vi "rsscope_core_global.vi"() -> ()   [LabVIEW 2018] (continued)
"Help"="Returns the cell count.\n\nAvailable Repeated Capabilities:\nSerialBus: SB1, SB2, SB3, SB4\r\n\nRemote-control command(s):\nBUS<m>:CMSB:FRAMe<n>:CCOunt?"}, {"Level"=5, "Class Only"=FALSE, "Identifier"="RSSCOPE_ATTR_PROTOCOL_MANCHESTER_NRZ_ADD_CELL", "Descriptive Name"="Protocol Manchester NRZ Add Cell", "Data Type"=4, "Command"="BUS{SerialBus}:CMSB:FRAM<Frame>:APP", "Access"=1, "Range Table"="", "Read Callback"="", "Write Callback"="rsscope_FormatManchesterNRZFrameRepCapEvent_WriteCallback.vi", "Supported Models"="", "Instrument Options"="K50", "Flags"=0, "Help"="Creates an empty cell description and adds it to the end of the active frame description.\n\nAvailable Repeated Capabilities:\nSerialBus: SB1, SB2, SB3, SB4\r\n\nRemote-control command(s):\nBUS<m>:CMSB:FRAMe<n>:APPend"}, {"Level"=5, "Class Only"=FALSE, "Identifier"="RSSCOPE_ATTR_PROTOCOL_MANCHESTER_NRZ_CELL_NAME", "Descriptive Name"="Protocol Manchester NRZ Cell Name", "Data Type"=2, "Command"="BUS{SerialBus}:CMSB:FRAM<Frame>:CELL<Cell>:NAME", "Access"=2, "Range Table"="", "Read Callback"="rsscope_FormatManchesterNRZFrameRepCapString_ReadCallback.vi", "Write Callback"="rsscope_FormatManchesterNRZFrameRepCapString_WriteCallback.vi", "Supported Models"="", "Instrument Options"="K50", "Flags"=0, "Help"="Enables the user to set a cell name within a frame. Names do not have to be unique, they are just for user support.\n\nAvailable Repeated Capabilities:\nSerialBus: SB1, SB2, SB3, SB4\r\n\nRemote-control command(s):\nBUS<m>:CMSB:FRAMe<n>:CELL<o>:NAME"}, {"Level"=5, "Class Only"=FALSE, "Identifier"="RSSCOPE_ATTR_PROTOCOL_MANCHESTER_NRZ_CELL_BIT_COUNT", "Descriptive Name"="Protocol Manchester NRZ Cell Bit Count", "Data Type"=0, "Command"="BUS{SerialBus}:CMSB:FRAM<Frame>:CELL<Cell>:BITC", "Access"=2, "Range Table"="RsScope_rngManchesterNRZCellBitCount", "Read Callback"="rsscope_FormatManchesterNRZFrameRepCapInt32_ReadCallback.vi", "Write Callback"="rsscope_FormatManchesterNRZFrameRepCapInt32_WriteCallback.vi", "Supported Models"="", "Instrument Options"="K50", "Flags"=0, "Help"="Sets the bit count of a cell, hence its length. Based upon the lengths of the previous cells, this also defines the position of the cell start and end within a frame.\n\nAvailable Repeated Capabilities:\nSerialBus: SB1, SB2, SB3, SB4\r\n\nRemote-control command(s):\nBUS<m>:CMSB:FRAMe<n>:CELL<o>:BITCount"}, {"Level"=5, "Class Only"=FALSE, "Identifier"="RSSCOPE_ATTR_PROTOCOL_MANCHESTER_NRZ_CELL_CONDITION", "Descriptive Name"="Protocol Manchester NRZ Cell Condition", "Data Type"=2, "Command"="BUS{SerialBus}:CMSB:FRAM<Frame>:CELL<Cell>:COND", "Access"=2, "Range Table"="", "Read Callback"="rsscope_FormatManchesterNRZFrameRepCapString_ReadCallback.vi", "Write Callback"="rsscope_FormatManchesterNRZFrameRepCapString_WriteCallback.vi", "Supported Models"="", "Instrument Options"="K50", "Flags"=0, "Help"="Sets various operators for a cell, to identify, e.g., mandatory values such as a CRC checksum or an ID, that help to identify a frame. The implemented conditions and functionalities are the &apos;equal&apos; and &apos;array&apos; operators. The numeric format of the condition needs to be set according to RSSCOPE_ATTR_PROTOCOL_MANCHESTER_NRZ_CELL_FORMAT.\n\nAvailable Repeated Capabilities:\nSerialBus: SB1, SB2, SB3, SB4\r\n\nRemote-control command(s):\nBUS<m>:CMSB:FRAMe<n>:CELL<o>:CONDition"}, {"Level"=5, "Class Only"=FALSE, "Identifier"="RSSCOPE_ATTR_PROTOCOL_MANCHESTER_NRZ_CELL_FORMAT", "Descriptive Name"="Protocol Manchester NRZ Cell Format", "Data Type"=0, "Command"="BUS{SerialBus}:CMSB:FRAM<Frame>:CELL<Cell>:FORM", "Access"=2, "Range Table"="RsScope_rngNumericFormat", "Read Callback"="rsscope_FormatManchesterNRZFrameRepCapInt32_ReadCallback.vi", "Write Callback"="rsscope_FormatManchesterNRZFrameRepCapInt32_WriteCallback.vi", "Supported Models"="", "Instrument Options"="K50", "Flags"=0, "Help"="Selects the numeric data format for the RSSCOPE_ATTR_PROTOCOL_MANCHESTER_NRZ_CELL_CONDITION, as well as for the result and honeycomb display.\n\nAvailable Repeated Capabilities:\nSerialBus: SB1, SB2, SB3, SB4\r\n\nRemote-control command(s):\nBUS<m>:CMSB:FRAMe<n>:CELL<o>:FORMat"}, {"Level"=5, "Class Only"=FALSE, "Identifier"="RSSCOPE_ATTR_PROTOCOL_MANCHESTER_NRZ_CELL_BIT_ORDER", "Descriptive Name"="Protocol Manchester NRZ Cell Bit Order", "Data Type"=0, "Command"="BUS{SerialBus}:CMSB:FRAM<Frame>:CELL<Cell>:BIT", "Access"=2, "Range Table"="rsscope_rngBitOrder", "Read Callback"="rsscope_FormatManchesterNRZFrameRepCapInt32_ReadCallback.vi", "Write Callback"="rsscope_FormatManchesterNRZFrameRepCapInt32_WriteCallback.vi", "Supported Models"="", "Instrument Options"="K50", "Flags"=0, "Help"="Selects in which order the bits of a cell are evaluated, as well as presented in the results table and honeycomb display.\n\nAvailable Repeated Capabilities:\nSerialBus: SB1, SB2, SB3, SB4\r\n\nRemote-control command(s):\nBUS<m>:CMSB:FRAMe<n>:CELL<o>:BITorder"}, {"Level"=5, "Class Only"=FALSE, "Identifier"="RSSCOPE_ATTR_PROTOCOL_MANCHESTER_NRZ_CELL_COLOR", "Descriptive Name"="Protocol Manchester NRZ Cell Color", "Data Type"=0, "Command"="BUS{SerialBus}:CMSB:FRAM<Frame>:CELL<Cell>:COL", "Access"=2, "Range Table"="RsScope_rngCellColor", "Read Callback"="rsscope_FormatManchesterNRZFrameRepCapInt32_ReadCallback.vi", "Write Callback"="rsscope_FormatManchesterNRZFrameRepCapInt32_WriteCallback.vi", "Supported Models"="", "Instrument Options"="K50", "Flags"=0, "Help"="Selects a cell&apos;s color representation in the honeycomb display.\n\nAvailable Repeated Capabilities:\nSerialBus: SB1, SB2, SB3, SB4\r\n\nRemote-control command(s):\nBUS<m>:CMSB:FRAMe<n>:CELL<o>:COLor"}, {"Level"=5, "Class Only"=FALSE, "Identifier"="RSSCOPE_ATTR_PROTOCOL_MANCHESTER_NRZ_CELL_COLOR_CRGB", "Descriptive Name"="Protocol Manchester NRZ Cell Color CRGB", "Data Type"=5, "Command"="BUS{SerialBus}:CMSB:FRAM<Frame>:CELL<Cell>:CRGB", "Access"=2, "Range Table"="", "Read Callback"="rsscope_FormatManchesterNRZFrameRepCapInt64_ReadCallback.vi", "Write Callback"="rsscope_FormatManchesterNRZFrameRepCapInt64_WriteCallback.vi", "Supported Models"="", "Instrument Options"="K50", "Flags"=0, "Help"="Selects a cell&apos;s color representation in the honeycomb display. ARGB value of the color to be used for the table entry.\nARGB=<Opacity(alpha) value><red value><green value><blue value>, in decimal format.\n\nAvailable Repeated Capabilities:\nSerialBus: SB1, SB2, SB3, SB4\r\n\nRemote-control command(s):\nBUS<m>:CMSB:FRAMe<n>:CELL<o>:CRGB"}, {"Level"=5, "Class Only"=FALSE, "Identifier"="RSSCOPE_ATTR_PROTOCOL_MANCHESTER_NRZ_CELL_RESULT_COLUMN", "Descriptive Name"="Protocol Manchester NRZ Cell Result Column", "Data Type"=0, "Command"="BUS{SerialBus}:CMSB:FRAM<Frame>:CELL<Cell>:CLMN", "Access"=2, "Range Table"="RsScope_rngCellResultColumn", "Read Callback"="rsscope_FormatManchesterNRZFrameRepCapInt32_ReadCallback.vi", "Write Callback"="rsscope_FormatManchesterNRZFrameRepCapInt32_WriteCallback.vi", "Supported Models"="", "Instrument Options"="K50", "Flags"=0, "Help"="Selects which cell shall be displayed in which result column of the decode table. The decode table supports three result columns, which have to be unique for each frame type. For different frame types, though, different result columns can be defined to display unrelated information.\n\nAvailable Repeated Capabilities:\nSerialBus: SB1, SB2, SB3, SB4\r\n\nRemote-control command(s):\nBUS<m>:CMSB:FRAMe<n>:CELL<o>:CLMN"}, {"Level"=3, "Class Only"=TRUE, "Identifier"="", "Descriptive Name"="Filter", "Data Type"=0, "Command"="", "Access"=0, "Range Table"="", "Read Callback"="", "Write Callback"="", "Supported Models"="", "Instrument Options"="", "Flags"=0, "Help"="Configures filtering of custom serial bus."}, {"Level"=4, "Class Only"=FALSE, "Identifier"="RSSCOPE_ATTR_PROTOCOL_MANCHESTER_NRZ_SELECTED_FIELD", "Descriptive Name"="Protocol Manchester NRZ Selected Field", "Data Type"=0, "Command"="", "Access"=2, "Range Table"="", "Read Callback"="", "Write Callback"="", "Supported Models"="", "Instrument Options"="", "Flags"=0, "Help"="Sets the selector for the Field repeated capability.\n\nAvailable Repeated Capabilities:\nNone\n\nRemote-control command(s):\n"}, {"Level"=4, "Class Only"=FALSE, "Identifier"="RSSCOPE_ATTR_PROTOCOL_MANCHESTER_NRZ_FILTER_ENABLED", "Descriptive Name"="Protocol Manchester NRZ Filter Enabled", "Data Type"=3, "Command"="BUS{SerialBus}:CMSB:FILT:ENAB", "Access"=2, "Range Table"="", "Read Callback"="", "Write Callback"="", "Supported Models"="", "Instrument Options"="K50", "Flags"=0, "Help"="Enables filtering for the custom serial bus.\n\nAvailable Repeated Capabilities:\nSerialBus: SB1, SB2, SB3, SB4\r\n\nRemote-control command(s):\nBUS<m>:CMSB:FILTer:ENABle"}, {"Level"=4, "Class Only"=FALSE, "Identifier"="RSSCOPE_ATTR_PROTOCOL_MANCHESTER_NRZ_FILTER_FRAME_FIELD_NUMERIC_ENABLED", "Descriptive Name"="Protocol Manchester NRZ Filter Frame Field Numeric Enabled", "Data Type"=3, "Command"="BUS{SerialBus}:CMSB:FILT:FRAM<Frame>:FLD<Field>:ENAB", "Access"=2, "Range Table"="", "Read Callback"="rsscope_FormatManchesterNRZFrameFieldRepCapBoolean_ReadCallback.vi", "Write Callback"="rsscope_FormatManchesterNRZFrameFieldRepCapBoolean_WriteCallback.vi", "Supported Models"="", "Instrument Options"="", "Flags"=0, "Help"="Enables or disables the specific field within the defined frame to be filtered.\n\nAvailable Repeated Capabilities:\nSerialBus: SB1, SB2, SB3, SB4\r\n\nRemote-control command(s):\nBUS<m>:CMSB:FILTer:FRAMe<Frame>:FLD<Field>:ENABle"}, {"Level"=4, "Class Only"=FALSE, "Identifier"="RSSCOPE_ATTR_PROTOCOL_MANCHESTER_NRZ_FILTER_FRAME_FIELD_BIT_STATE", "Descriptive Name"="Protocol Manchester NRZ Filter Frame Field Bit State", "Data Type"=0, "Command"="BUS{SerialBus}:CMSB:FILT:FRAM<Frame>:FLD<Field>:BIT", "Access"=2, "Range Table"="RsScope_rngBitState", "Read Callback"="rsscope_FormatManchesterNRZFrameFieldRepCapInt32_ReadCallback.vi", "Write Callback"="rsscope_FormatManchesterNRZFrameFieldRepCapInt32_WriteCallback.vi", "Supported Models"="", "Instrument Options"="", "Flags"=0, "Help"="Sets the bit state of a field to be filtered on that only consists of one bit.\n\nAvailable Repeated Capabilities:\nSerialBus: SB1, SB2, SB3, SB4\r\n\nRemote-control command(s):\nBUS<m>:CMSB:FILTer:FRAMe<n>:FLD<o>:BIT"}, {"Level"=4, "Class Only"=FALSE, "Identifier"="RSSCOPE_ATTR_PROTOCOL_MANCHESTER_NRZ_FILTER_FRAME_FIELD_DATA_PATTERN_CONDITION", "Descriptive Name"="Protocol Manchester NRZ Filter Frame Field Data Pattern Condition", "Data Type"=0, "Command"="BUS{SerialBus}:CMSB:FILT:FRAM<Frame>:FLD<Field>:DOP", "Access"=2, "Range Table"="rsscope_rngCustomSBCondition", "Read Callback"="rsscope_FormatManchesterNRZFrameFieldRepCapInt32_ReadCallback.vi", "Write Callback"="rsscope_FormatManchesterNRZFrameFieldRepCapInt32_WriteCallback.vi", "Supported Models"="", "Instrument Options"="", "Flags"=0, "Help"="Sets the operator for the data pattern.\n\nAvailable Repeated Capabilities:\nSerialBus: SB1, SB2, SB3, SB4\r\n\nRemote-control command(s):\nBUS<m>:CMSB:FILTer:FRAMe<n>:FLD<o>:DOPerator"}, {"Level"=4, "Class Only"=FALSE, "Identifier"="RSSCOPE_ATTR_PROTOCOL_MANCHESTER_NRZ_FILTER_FRAME_FIELD_DATA_PATTERN_MIN", "Descriptive Name"="Protocol Manchester NRZ Filter Frame Field Data Pattern Min", "Data Type"=6, "Command"="BUS{SerialBus}:CMSB:FILT:FRAM<Frame>:FLD<Field>:DMIN", "Access"=2, "Range Table"="", "Read Callback"="rsscope_FormatManchesterNRZFrameFieldRepCapRawString_ReadCallback.vi", "Write Callback"="rsscope_FormatManchesterNRZFrameFieldRepCapRawString_WriteCallback.vi", "Supported Models"="", "Instrument Options"="", "Flags"=0, "Help"="Specifies the data pattern, or sets the start value of a data pattern range.\n\nAvailable Repeated Capabilities:\nSerialBus: SB1, SB2, SB3, SB4\r\n\nRemote-control command(s):\nBUS<m>:CMSB:FILTer:FRAMe<n>:FLD<o>:DMIN"}, {"Level"=4, "Class Only"=FALSE, "Identifier"="RSSCOPE_ATTR_PROTOCOL_MANCHESTER_NRZ_FILTER_FRAME_FIELD_DATA_PATTERN_MAX", "Descriptive Name"="Protocol Manchester NRZ Filter Frame Field Data Pattern Max", "Data Type"=6, "Command"="BUS{SerialBus}:CMSB:FILT:FRAM<Frame>:FLD<Field>:DMAX", "Access"=2, "Range Table"="", "Read Callback"="rsscope_FormatManchesterNRZFrameFieldRepCapRawString_ReadCallback.vi", "Write Callback"="rsscope_FormatManchesterNRZFrameFieldRepCapRawString_WriteCallback.vi", "Supported Models"="", "Instrument Options"="", "Flags"=0, "Help"="Sets the end value of a data pattern range if RSSCOPE_ATTR_PROTOCOL_MANCHESTER_NRZ_FILTER_FRAME_FIELD_DATA_PATTERN_CONDITION is set to In Range or Out Of Range.\n\nAvailable Repeated Capabilities:\nSerialBus: SB1, SB2, SB3, SB4\r\n\nRemote-control command(s):\nBUS<m>:CMSB:FILTer:FRAMe<n>:FLD<o>:DMAX"}, {"Level"=4, "Class Only"=FALSE, "Identifier"="RSSCOPE_ATTR_PROTOCOL_MANCHESTER_NRZ_FILTER_FRAME_FIELD_INDEX_PATTERN_CONDITION", "Descriptive Name"="Protocol Manchester NRZ Filter Frame Field Index Pattern Condition", "Data Type"=0, "Command"="BUS{SerialBus}:CMSB:FILT:FRAM<Frame>:FLD<Field>:IOP", "Access"=2, "Range Table"="rsscope_rngCustomSBCondition", "Read Callback"="rsscope_FormatManchesterNRZFrameFieldRepCapInt32_ReadCallback.vi", "Write Callback"="rsscope_FormatManchesterNRZFrameFieldRepCapInt32_WriteCallback.vi", "Supported Models"="", "Instrument Options"="", "Flags"=0, "Help"="Sets the operator for the index in the selected field of the selected frame.\n\nAvailable Repeated Capabilities:\nSerialBus: SB1, SB2, SB3, SB4\r\n\nRemote-control command(s):\nBUS<m>:CMSB:FILTer:FRAMe<n>:FLD<o>:IOPerator"}, {"Level"=4, "Class Only"=FALSE, "Identifier"="RSSCOPE_ATTR_PROTOCOL_MANCHESTER_NRZ_FILTER_FRAME_FIELD_INDEX_PATTERN_MIN", "Descriptive Name"="Protocol Manchester NRZ Filter Frame Field Index Pattern Min", "Data Type"=6, "Command"="BUS{SerialBus}:CMSB:FILT:FRAM<Frame>:FLD<Field>:IMIN", "Access"=2, "Range Table"="", "Read Callback"="rsscope_FormatManchesterNRZFrameFieldRepCapRawString_ReadCallback.vi", "Write Callback"="rsscope_FormatManchesterNRZFrameFieldRepCapRawString_WriteCallback.vi", "Supported Models"="", "Instrument Options"="", "Flags"=0, "Help"="Specifies the index, or sets the start value of an index range.\n\nAvailable Repeated Capabilities:\nSerialBus: SB1, SB2, SB3, SB4\r\n\nRemote-control command(s):\nBUS<m>:CMSB:FILTer:FRAMe<n>:FLD<o>:IMIN"}, {"Level"=4, "Class Only"=FALSE, "Identifier"="RSSCOPE_ATTR_PROTOCOL_MANCHESTER_NRZ_FILTER_FRAME_FIELD_INDEX_PATTERN_MAX", "Descriptive Name"="Protocol Manchester NRZ Filter Frame Field Index Pattern Max", "Data Type"=6, "Command"="BUS{SerialBus}:CMSB:FILT:FRAM<Frame>:FLD<Field>:IMAX", "Access"=2, "Range Table"="", "Read Callback"="rsscope_FormatManchesterNRZFrameFieldRepCapRawString_ReadCallback.vi", "Write Callback"="rsscope_FormatManchesterNRZFrameFieldRepCapRawString_WriteCallback.vi", "Supported Models"="", "Instrument Options"="", "Flags"=0, "Help"="Sets the end value of a index pattern range if RSSCOPE_ATTR_PROTOCOL_MANCHESTER_NRZ_FILTER_FRAME_FIELD_INDEX_PATTERN_CONDITION is set to In Range or Out Of Range.\n\nAvailable Repeated Capabilities:\nSerialBus: SB1, SB2, SB3, SB4\r\n\nRemote-control command(s):\nBUS<m>:CMSB:FILTer:FRAMe<n>:FLD<o>:IMAX"}, {"Level"=3, "Class Only"=TRUE, "Identifier"="", "Descriptive Name"="Decoding Results", "Data Type"=0, "Command"="", "Access"=0, "Range Table"="", "Read Callback"="", "Write Callback"="", "Supported Models"="", "Instrument Options"="", "Flags"=0, "Help"="Returns the decoding results."}, {"Level"=4, "Class Only"=FALSE, "Identifier"="RSSCOPE_ATTR_PROTOCOL_MANCHESTER_NRZ_RESULT_COUNT", "Descriptive Name"="Protocol Manchester NRZ Result Count", "Data Type"=0, "Command"="BUS{SerialBus}:CMSB:RCO?", "Access"=0, "Range Table"="", "Read Callback"="", "Write Callback"="", "Supported Models"="", "Instrument Options"="K50", "Flags"=0, "Help"="Returns the count number of decoded result frames in a custom serial bus waveform.\n\nAvailable Repeated Capabilities:\nSerialBus: SB1, SB2, SB3, SB4\r\n\nRemote-control command(s):\nBUS<m>:CMSB:RCOunt?"}, {"Level"=2, "Class Only"=TRUE, "Identifier"="", "Descriptive Name"="EbTb", "Data Type"=0, "Command"="", "Access"=0, "Range Table"="", "Read Callback"="", "Write Callback"="", "Supported Models"="", "Instrument Options"="", "Flags"=0, "Help"="The 8b/10b (Option R&S RTO-K52) coding scheme is used for high-speed serial data transmission, used by different standards, like fibre channel, PCIe, DVI and USB 3.0. Also the MIPI UniPro M-PHY interface in smartphones as well as display interfaces such as HDMI use 8b/10b encoding, as do base stations based on the Common Public Radio Interface (CPRI)."}, {"Level"=3, "Class Only"=FALSE, "Identifier"="RSSCOPE_ATTR_PROTOCOLS_EBTB_SIGNAL_TYPE", "Descriptive Name"="Protocols EbTb Signal Type", "Data Type"=0, "Command"="BUS{SerialBus}:EBTB:TYPE", "Access"=2, "Range Table"="RsScope_rngSignalType", "Read Callback"="", "Write Callback"="", "Supported Models"="", "Instrument Options"="K52", "Flags"=0, "Help"="Selects the signal type that is used for the decoding. You can choose between a differential and single-ended signal.\n\nAvailable Repeated Capabilities:\nSerialBus: SB1, SB2, SB3, SB4\r\n\nRemote-control command(s):\nBUS<m>:EBTB:TYPE"}, {"Level"=3, "Class Only"=FALSE, "Identifier"="RSSCOPE_ATTR_PROTOCOLS_EBTB_DIFFERENTIAL_SOURCE", "Descriptive Name"="Protocols EbTb Differential Source", "Data Type"=0, "Command"="BUS{SerialBus}:EBTB:DIFF:SOUR", "Access"=2, "Range Table"="rsscope_rngWaveformParameter", "Read Callback"="", "Write Callback"="", "Supported Models"="", "Instrument Options"="K52", "Flags"=0, "Help"="Selects the source of the provided differential signal, if 'Signal type' > 'Differential'.\n\nAvailable Repeated Capabilities:\nSerialBus: SB1, SB2, SB3, SB4\r\n\nRemote-control command(s):\nBUS<m>:EBTB:DIFFerential:SOURce"}, {"Level"=3, "Class Only"=FALSE, "Identifier"="RSSCOPE_ATTR_PROTOCOLS_EBTB_D_PLUS_SOURCE", "Descriptive Name"="Protocols EbTb D Plus Source", "Data Type"=0, "Command"="BUS{SerialBus}:EBTB:DPL:SOUR", "Access"=2, "Range Table"="rsscope_rngWaveformParameter", "Read Callback"="", "Write Callback"="", "Supported Models"="", "Instrument Options"="K52", "Flags"=0, "Help"="Selects the D+ source of the provided single-ended signal, if 'Signal type' > 'Single.\n\nAvailable Repeated Capabilities:\nSerialBus: SB1, SB2, SB3, SB4\r\n\nRemote-control command(s):\nBUS<m>:EBTB:DPLus:SOURce"}, {"Level"=3, "Class Only"=FALSE, "Identifier"="RSSCOPE_ATTR_PROTOCOLS_EBTB_D_MINUS_SOURCE", "Descriptive Name"="Protocols EbTb D Minus Source", "Data Type"=0, "Command"="BUS{SerialBus}:EBTB:DMIN:SOUR", "Access"=2, "Range Table"="rsscope_rngWaveformParameter", "Read Callback"="", "Write Callback"="", "Supported Models"="", "Instrument Options"="K52", "Flags"=0, "Help"="Selects the D- source of the provided single ended signal, if 'Signal type' > 'Single\n\nAvailable Repeated Capabilities:\nSerialBus: SB1, SB2, SB3, SB4\r\n\nRemote-control command(s):\nBUS<m>:EBTB:DMINus:SOURce"}, {"Level"=3, "Class Only"=FALSE, "Identifier"="RSSCOPE_ATTR_PROTOCOLS_EBTB_FULL_AUTOSET", "Descriptive Name"="Protocols EbTb Full Autoset", "Data Type"=4, "Command"="BUS{SerialBus}:EBTB:FAUT", "Access"=1, "Range Table"="", "Read Callback"="", "Write Callback"="", "Supported Models"="", "Instrument Options"="K52", "Flags"=0, "Help"="Starts software algorithms for determining the signal threshold levels and bitrate.\n\nAvailable Repeated Capabilities:\nSerialBus: SB1, SB2, SB3, SB4\r\n\nRemote-control command(s):\nBUS<m>:EBTB:FAUToscale"}, {"Level"=3, "Class Only"=FALSE, "Identifier"="RSSCOPE_ATTR_PROTOCOLS_EBTB_DIFFERENTIAL_THRESHOLD_HIGH", "Descriptive Name"="Protocols EbTb Differential Threshold High", "Data Type"=1, "Command"="BUS{SerialBus}:EBTB:DIFF:THRH", "Access"=2, "Range Table"="RsScope_rngEbTbThreshold", "Read Callback"="", "Write Callback"="", "Supported Models"="", "Instrument Options"="K52", "Flags"=0, "Help"="Sets the threshold high of the signal, if &apos;Signal type&apos; > &apos;Differential&apos;.\n\nAvailable Repeated Capabilities:\nSerialBus: SB1, SB2, SB3, SB4\r\n\nRemote-control command(s):\nBUS<m>:EBTB:DIFFerential:THRHigh"}, {"Level"=3, "Class Only"=FALSE, "Identifier"="RSSCOPE_ATTR_PROTOCOLS_EBTB_DIFFERENTIAL_THRESHOLD_LOW", "Descriptive Name"="Protocols EbTb Differential Threshold Low", "Data Type"=1, "Command"="BUS{SerialBus}:EBTB:DIFF:THRL", "Access"=2, "Range Table"="RsScope_rngEbTbThreshold", "Read Callback"="", "Write Callback"="", "Supported Models"="", "Instrument Options"="K52", "Flags"=0, "Help"="Sets the threshold low of the signal, if &apos;Signal type&apos; > &apos;Differential&apos;.\n\nAvailable Repeated Capabilities:\nSerialBus: SB1, SB2, SB3, SB4\r\n\nRemote-control command(s):\nBUS<m>:EBTB:DIFFerential:THRLow"}, {"Level"=3, "Class Only"=FALSE, "Identifier"="RSSCOPE_ATTR_PROTOCOLS_EBTB_THRESHOLD_D_PLUS", "Descriptive Name"="Protocols EbTb Threshold D Plus", "Data Type"=1, "Command"="BUS{SerialBus}:EBTB:DPL:THR", "Access"=2, "Range Table"="RsScope_rngEbTbThreshold", "Read Callback"="", "Write Callback"="", "Supported Models"="", "Instrument Options"="K52", "Flags"=0, "Help"="Sets the high threshold (D+) of the signal, if &apos;Signal type&apos; > &apos;Single&apos;.\n\nAvailable Repeated Capabilities:\nSerialBus: SB1, SB2, SB3, SB4\r\n\nRemote-control command(s):\nBUS<m>:EBTB:DPLus:THReshold"}, {"Level"=3, "Class Only"=FALSE, "Identifier"="RSSCOPE_ATTR_PROTOCOLS_EBTB_THRESHOLD_D_MINUS", "Descriptive Name"="Protocols EbTb Threshold D Minus", "Data Type"=1, "Command"="BUS{SerialBus}:EBTB:DMIN:THR", "Access"=2, "Range Table"="RsScope_rngEbTbThreshold", "Read Callback"="", "Write Callback"="", "Supported Models"="", "Instrument Options"="K52", "Flags"=0, "Help"="Sets the low threshold (D-) of the signal, if &apos;Signal type&apos; > &apos;Single&apos;.\n\nAvailable Repeated Capabilities:\nSerialBus: SB1, SB2, SB3, SB4\r\n\nRemote-control command(s):\nBUS<m>:EBTB:DMINus:THReshold"}, {"Level"=3, "Class Only"=FALSE, "Identifier"="RSSCOPE_ATTR_PROTOCOLS_EBTB_BITRATE", "Descriptive Name"="Protocols EbTb Bitrate", "Data Type"=1, "Command"="BUS{SerialBus}:EBTB:BITR", "Access"=2, "Range Table"="RsScope_rngEbTbBitrate", "Read Callback"="", "Write Callback"="", "Supported Models"="", "Instrument Options"="K52", "Flags"=0, "Help"="Sets the number of transmitted bits per second.\n\nAvailable Repeated Capabilities:\nSerialBus: SB1, SB2, SB3, SB4\r\n\nRemote-control command(s):\nBUS<m>:EBTB:BITRate"}, {"Level"=3, "Class Only"=FALSE, "Identifier"="RSSCOPE_ATTR_PROTOCOLS_EBTB_BITRATE_DETERMINATION", "Descriptive Name"="Protocols EbTb Bitrate Determination", "Data Type"=4, "Command"="BUS{SerialBus}:EBTB:BITD", "Access"=1, "Range Table"="", "Read Callback"="", "Write Callback"="", "Supported Models"="", "Instrument Options"="K52", "Flags"=0, "Help"="Starts a software algorithm for the automatic determination of the bitrate.\n\nAvailable Repeated Capabilities:\nSerialBus: SB1, SB2, SB3, SB4\r\n\nRemote-control command(s):\nBUS<m>:EBTB:BITDetermi"}, {"Level"=3, "Class Only"=FALSE, "Identifier"="RSSCOPE_ATTR_PROTOCOLS_EBTB_ESTIMATED_BITRATE", "Descriptive Name"="Protocols EbTb Estimated Bitrate", "Data Type"=1, "Command"="BUS{SerialBus}:EBTB:EBTR?", "Access"=0, "Range Table"="", "Read Callback"="", "Write Callback"="", "Supported Models"="", "Instrument Options"="K52", "Flags"=0, "Help"="Queries the estimated bitrate value.\n\nAvailable Repeated Capabilities:\nSerialBus: SB1, SB2, SB3, SB4\r\n\nRemote-control command(s):\nBUS<m>:EBTB:EBTRate?"}, {"Level"=3, "Class Only"=FALSE, "Identifier"="RSSCOPE_ATTR_PROTOCOLS_EBTB_SW_CDR_BITRATE", "Descriptive Name"="Protocols EbTb SW CDR Bitrate", "Data Type"=3, "Command"="BUS{SerialBus}:EBTB:ACT", "Access"=2, "Range Table"="", "Read Callback"="", "Write Callback"="", "Supported Models"="", "Instrument Options"="K52", "Flags"=0, "Help"="Disables the automatic software birtate determination.\n\nAvailable Repeated Capabilities:\nSerialBus: SB1, SB2, SB3, SB4\r\n\nRemote-control command(s):\nBUS<m>:EBTB:ACTestimate"}, {"Level"=3, "Class Only"=FALSE, "Identifier"="RSSCOPE_ATTR_PROTOCOLS_EBTB_SYNC_SYMBOL", "Descriptive Name"="Protocols EbTb Sync Symbol", "Data Type"=0, "Command"="BUS{SerialBus}:EBTB:SYNC", "Access"=2, "Range Table"="RsScope_rngEbTbSyncSymbol", "Read Callback"="", "Write Callback"="", "Supported Models"="", "Instrument Options"="K52", "Flags"=0, "Help"="Selects the sync symbol, a control symbol used for low level control functions. You can select one of the comma control symbols (K28.1, K28.5, K28.7) used for synchronisation or you can enter a pattern.\n\nAvailable Repeated Capabilities:\nSerialBus: SB1, SB2, SB3, SB4\r\n\nRemote-control command(s):\nBUS<m>:EBTB:SYNC"}, {"Level"=3, "Class Only"=FALSE, "Identifier"="RSSCOPE_ATTR_PROTOCOLS_EBTB_PATTERN", "Descriptive Name"="Protocols EbTb Pattern", "Data Type"=0, "Command"="BUS{SerialBus}:EBTB:FCSY", "Access"=2, "Range Table"="", "Read Callback"="", "Write Callback"="", "Supported Models"="", "Instrument Options"="K52", "Flags"=0, "Help"="Selects a pattern that serves as a sync symbol.\n\nAvailable Repeated Capabilities:\nSerialBus: SB1, SB2, SB3, SB4\r\n\nRemote-control command(s):\nBUS<m>:EBTB:FCSY"}, {"Level"=3, "Class Only"=FALSE, "Identifier"="RSSCOPE_ATTR_PROTOCOLS_EBTB_SECOND_PATTERN_ENABLED", "Descriptive Name"="Protocols EbTb Second Pattern Enabled", "Data Type"=3, "Command"="BUS{SerialBus}:EBTB:USCS", "Access"=2, "Range Table"="", "Read Callback"="", "Write Callback"="", "Supported Models"="", "Instrument Options"="K52", "Flags"=0, "Help"="Selects whether the second pattern is enabled.\n\nAvailable Repeated Capabilities:\nSerialBus: SB1, SB2, SB3, SB4\r\n\nRemote-control command(s):\nBUS<m>:EBTB:USCS"}, {"Level"=3, "Class Only"=FALSE, "Identifier"="RSSCOPE_ATTR_PROTOCOLS_EBTB_SECOND_PATTERN", "Descriptive Name"="Protocols EbTb Second Pattern", "Data Type"=0, "Command"="BUS{SerialBus}:EBTB:SCSY", "Access"=2, "Range Table"="", "Read Callback"="", "Write Callback"="", "Supported Models"="", "Instrument Options"="K52", "Flags"=0, "Help"="Sets the value for the second pattern.\n\nAvailable Repeated Capabilities:\nSerialBus: SB1, SB2, SB3, SB4\r\n\nRemote-control command(s):\nBUS<m>:EBTB:SCSY"}, {"Level"=3, "Class Only"=FALSE, "Identifier"="RSSCOPE_ATTR_PROTOCOLS_EBTB_DISPLAY_FORMAT", "Descriptive Name"="Protocols EbTb Display Format", "Data Type"=0, "Command"="BUS{SerialBus}:EBTB:DISF", "Access"=2, "Range Table"="RsScope_rngEbTbDisplayFormat", "Read Callback"="", "Write Callback"="", "Supported Models"="", "Instrument Options"="K52", "Flags"=0, "Help"="Selects the display format for the results in the decode table.\n\nAvailable Repeated Capabilities:\nSerialBus: SB1, SB2, SB3, SB4\r\n\nRemote-control command(s):\nBUS<m>:EBTB:DISF"}, {"Level"=3, "Class Only"=TRUE, "Identifier"="", "Descriptive Name"="Decoding Results", "Data Type"=0, "Command"="", "Access"=0, "Range Table"="", "Read Callback"="", "Write Callback"="", "Supported Models"="", "Instrument Options"="", "Flags"=0, "Help"="Returns the decoding results."}, {"Level"=4, "Class Only"=FALSE, "Identifier"="RSSCOPE_ATTR_PROTOCOL_EBTB_SYMBOL_COUNT", "Descriptive Name"="Protocol EbTb Symbol Count", "Data Type"=0, "Command"="BUS{SerialBus}:EBTB:SCO?", "Access"=0, "Range Table"="", "Read Callback"="", "Write Callback"="", "Supported Models"="", "Instrument Options"="K52", "Flags"=0, "Help"="Returns the symbol count for the selected serial bus, i.e. the number of symbols in the present acquisition.\n\nAvailable Repeated Capabilities:\nSerialBus: SB1, SB2, SB3, SB4\r\n\nRemote-control command(s):\nBUS<m>:EBTB:SCOunt?"}, {"Level"=2, "Class Only"=TRUE, "Identifier"="", "Descriptive Name"="SENT", "Data Type"=0, "Command"="", "Access"=0, "Range Table"="", "Read Callback"="", "Write Callback"="", "Supported Models"="", "Instrument Options"="", "Flags"=0, "Help"="SENT (Single Ended Nibble Transmission, R&S RTO-K10 option) is a serial transmission interface protocol originally specified for the communication of sensors and control units in automotive electronics."}, {"Level"=3, "Class Only"=FALSE, "Identifier"="RSSCOPE_ATTR_PROTOCOL_SENT_DATA_SOURCE", "Descriptive Name"="Protocol SENT Data Source", "Data Type"=0, "Command"="BUS{SerialBus}:SENT:DATA:SOUR", "Access"=2, "Range Table"="rsscope_rngProtocolWaveformSource", "Read Callback"="", "Write Callback"="", "Supported Models"="", "Instrument Options"="K10", "Flags"=0, "Help"="Selects the source of the data line.\n\nAvailable Repeated Capabilities:\nSerialBus: SB1, SB2, SB3, SB4\r\n\nRemote-control command(s):\nBUS<m>:SENT:DATA:SOURce"}, {"Level"=3, "Class Only"=FALSE, "Identifier"="RSSCOPE_ATTR_PROTOCOL_SENT_THRESHOLD", "Descriptive Name"="Protocol SENT Threshold", "Data Type"=1, "Command"="BUS{SerialBus}:SENT:DATA:THR", "Access"=2, "Range Table"="RsScope_rngSENTThreshold", "Read Callback"="", "Write Callback"="", "Supported Models"="", "Instrument Options"="K10", "Flags"=0, "Help"="Sets a user-defined threshold value.\n\nAvailable Repeated Capabilities:\nSerialBus: SB1, SB2, SB3, SB4\r\n\nRemote-control command(s):\nBUS<m>:SENT:DATA:THReshold"}, {"Level"=3, "Class Only"=FALSE, "Identifier"="RSSCOPE_ATTR_PROTOCOL_SENT_TECHNOLOGY", "Descriptive Name"="Protocol SENT Technology", "Data Type"=0, "Command"="BUS{SerialBus}:SENT:TECH", "Access"=2, "Range Table"="RsScope_rngSENTTechnology", "Read Callback"="", "Write Callback"="", "Supported Models"="", "Instrument Options"="K10", "Flags"=0, "Help"="Selects the threshold voltage.\n\nAvailable Repeated Capabilities:\nSerialBus: SB1, SB2, SB3, SB4\r\n\nRemote-control command(s):\nBUS<m>:SENT:TECHnology"}, {"Level"=3, "Class Only"=FALSE, "Identifier"="RSSCOPE_ATTR_PROTOCOL_SENT_CLOCK_PERIOD", "Descriptive Name"="Protocol SENT Clock Period", "Data Type"=1, "Command"="BUS{SerialBus}:SENT:CLKP", "Access"=2, "Range Table"="RsScope_rngSENTClockPeriod", "Read Callback"="", "Write Callback"="", "Supported Models"="", "Instrument Options"="K10", "Flags"=0, "Help"="Sets the nominal clock period (clock tick).\n\nAvailable Repeated Capabilities:\nSerialBus: SB1, SB2, SB3, SB4\r\n\nRemote-control command(s):\nBUS<m>:SENT:CLKPeriod"}, {"Level"=3, "Class Only"=FALSE, "Identifier"="RSSCOPE_ATTR_PROTOCOL_SENT_CLOCK_TOLERANCE", "Descriptive Name"="Protocol SENT Clock Tolerance", "Data Type"=1, "Command"="BUS{SerialBus}:SENT:CLKT", "Access"=2, "Range Table"="RsScope_rngSENTClockTolerance", "Read Callback"="", "Write Callback"="", "Supported Models"="", "Instrument Options"="K10", "Flags"=0, "Help"="Specifies a tolerated deviation of the clock.\n\nAvailable Repeated Capabilities:\nSerialBus: SB1, SB2, SB3, SB4\r\n\nRemote-control command(s):\nBUS<m>:SENT:CLKTolerance"}, {"Level"=3, "Class Only"=FALSE, "Identifier"="RSSCOPE_ATTR_PROTOCOL_SENT_DATA_NIBBLES", "Descriptive Name"="Protocol SENT Data Nibbles", "Data Type"=0, "Command"="BUS{SerialBus}:SENT:DNIB", "Access"=2, "Range Table"="RsScope_rngSENTDataNibbles", "Read Callback"="", "Write Callback"="", "Supported Models"="", "Instrument Options"="K10", "Flags"=0, "Help"="Sets the number of data nibbles for a transmission sequence.\n\nAvailable Repeated Capabilities:\nSerialBus: SB1, SB2, SB3, SB4\r\n\nRemote-control command(s):\nBUS<m>:SENT:DNIBbles"}, {"Level"=3, "Class Only"=FALSE, "Identifier"="RSSCOPE_ATTR_PROTOCOL_SENT_SERIAL_FORMAT", "Descriptive Name"="Protocol SENT Serial Format", "Data Type"=0, "Command"="BUS{SerialBus}:SENT:SFOR", "Access"=2, "Range Table"="RsScope_rngSENTSerialFormat", "Read Callback"="", "Write Callback"="", "Supported Models"="", "Instrument Options"="K10", "Flags"=0, "Help"="Selects the serial message format.\n\nAvailable Repeated Capabilities:\nSerialBus: SB1, SB2, SB3, SB4\r\n\nRemote-control command(s):\nBUS<m>:SENT:SFORmat"}, {"Level"=3, "Class Only"=FALSE, "Identifier"="RSSCOPE_ATTR_PROTOCOL_SENT_CRC_VERSION", "Descriptive Name"="Protocol SENT CRC Version", "Data Type"=0, "Command"="BUS{SerialBus}:SENT:CRCV", "Access"=2, "Range Table"="RsScope_rngSENTCRCVersion", "Read Callback"="", "Write Callback"="", "Supported Models"="", "Instrument Options"="K10", "Flags"=0, "Help"="Selects the calculaction method for the cyclic redundancy check (CRC).\n\nAvailable Repeated Capabilities:\nSerialBus: SB1, SB2, SB3, SB4\r\n\nRemote-control command(s):\nBUS<m>:SENT:CRCVersion"}, {"Level"=3, "Class Only"=FALSE, "Identifier"="RSSCOPE_ATTR_PROTOCOL_SENT_CRC_CALCULATION", "Descriptive Name"="Protocol SENT CRC Calculation", "Data Type"=0, "Command"="BUS{SerialBus}:SENT:CRCM", "Access"=2, "Range Table"="RsScope_rngSENTCRCMethod", "Read Callback"="", "Write Callback"="", "Supported Models"="", "Instrument Options"="K10", "Flags"=0, "Help"="Selects the method for CRC calculation. SENT CRC calculates the checksum over all nibbles except the communication and\nstatus nibble.\n\nAvailable Repeated Capabilities:\nSerialBus: SB1, SB2, SB3, SB4\r\n\nRemote-control command(s):\nBUS<m>:SENT:CRCMethod"}, {"Level"=3, "Class Only"=FALSE, "Identifier"="RSSCOPE_ATTR_PROTOCOL_SENT_PAUSE_PULSE", "Descriptive Name"="Protocol SENT Pause Pulse", "Data Type"=0, "Command"="BUS{SerialBus}:SENT:PPUL", "Access"=2, "Range Table"="RsScope_rngSENTPausePulse", "Read Callback"="", "Write Callback"="", "Supported Models"="", "Instrument Options"="K10", "Flags"=0, "Help"="Determines wether a pause pulse is part of the SENT transmission sequence.\n\nAvailable Repeated Capabilities:\nSerialBus: SB1, SB2, SB3, SB4\r\n\nRemote-control command(s):\nBUS<m>:SENT:PPULse"}, {"Level"=3, "Class Only"=FALSE, "Identifier"="RSSCOPE_ATTR_PROTOCOL_SENT_FRAME_LENGTH", "Descriptive Name"="Protocol SENT Frame Length", "Data Type"=0, "Command"="BUS{SerialBus}:SENT:PPFL", "Access"=2, "Range Table"="RsScope_rngSENTFrameLength", "Read Callback"="", "Write Callback"="", "Supported Models"="", "Instrument Options"="K10", "Flags"=0, "Help"="Determines the frame length in terms of ticks. The dialog displays this settings parameter, if the signal has a constant frame length.\n\nAvailable Repeated Capabilities:\nSerialBus: SB1, SB2, SB3, SB4\r\n\nRemote-control command(s):\nBUS<m>:SENT:PPFLength"}, {"Level"=3, "Class Only"=FALSE, "Identifier"="RSSCOPE_ATTR_PROTOCOL_SENT_RESULT_DISPLAY", "Descriptive Name"="Protocol SENT Result Display", "Data Type"=0, "Command"="BUS{SerialBus}:SENT:RDSL", "Access"=2, "Range Table"="RsScope_rngSENTResultDisplay", "Read Callback"="", "Write Callback"="", "Supported Models"="", "Instrument Options"="K10", "Flags"=0, "Help"="Selects the results to be displayed.\n\nAvailable Repeated Capabilities:\nSerialBus: SB1, SB2, SB3, SB4\r\n\nRemote-control command(s):\nBUS<m>:SENT:RDSL"}, {"Level"=3, "Class Only"=TRUE, "Identifier"="", "Descriptive Name"="Decoding Results", "Data Type"=0, "Command"="", "Access"=0, "Range Table"="", "Read Callback"="", "Write Callback"="", "Supported Models"="", "Instrument Options"="", "Flags"=0, "Help"="Returns the decoding results."}, {"Level"=4, "Class Only"=FALSE, "Identifier"="RSSCOPE_ATTR_PROTOCOL_SENT_FRAME_COUNT", "Descriptive Name"="Protocol SENT Frame Count", "Data Type"=0, "Command"="BUS{SerialBus}:SENT:FCO?", "Access"=0, "Range Table"="", "Read Callback"="", "Write Callback"="", "Supported Models"="", "Instrument Options"="K10", "Flags"=0, "Help"="Returns the number of decoded frames of the acquisition.\n\nAvailable Repeated Capabilities:\nSerialBus: SB1, SB2, SB3, SB4\r\n\nRemote-control command(s):\nBUS<m>:SENT:FCOunt?"}, {"Level"=2, "Class Only"=TRUE, "Identifier"="", "Descriptive Name"="D-PHY", "Data Type"=0, "Command"="", "Access"=0, "Range Table"="", "Read Callback"="", "Write Callback"="", "Supported Models"="", "Instrument Options"="", "Flags"=0, "Help"="The D-PHY is a specification developed by the Mobile Industry Processor Interface (MIPI) alliance as a standard for the communication of high-speed components, like cameras and displays, within mobile devices."}, {"Level"=3, "Class Only"=FALSE, "Identifier"="RSSCOPE_ATTR_PROTOCOL_DPHY_VARIANT", "Descriptive Name"="Protocol DPHY Variant", "Data Type"=0, "Command"="BUS{SerialBus}:DPHY:VAR", "Access"=2, "Range Table"="RsScope_rngDPHYVariant", "Read Callback"="", "Write Callback"="", "Supported Models"="", "Instrument Options"="K42", "Flags"=0, "Help"="Selects the protocol running on the interface. You can select between the Display Serial Interface (DSI) and Camera Serial Interface (CSI-2).\n\nAvailable Repeated Capabilities:\nSerialBus: SB1, SB2, SB3, SB4\r\n\nRemote-control command(s):\nBUS<m>:DPHY:VARiant"}, {"Level"=3, "Class Only"=FALSE, "Identifier"="RSSCOPE_ATTR_PROTOCOL_DPHY_PHYSICAL_CONFIGURATION", "Descriptive Name"="Protocol DPHY Physical Configuration", "Data Type"=0, "Command"="BUS{SerialBus}:DPHY:CONF", "Access"=2, "Range Table"="RsScope_rngProtocolDPHYPhysicalConfiguration", "Read Callback"="", "Write Callback"="", "Supported Models"="", "Instrument Options"="K42", "Flags"=0, "Help"="Sets the number of data lanes and if the clock lane and low power are available.\n\nAvailable Repeated Capabilities:\nSerialBus: SB1, SB2, SB3, SB4\r\n\nRemote-control command(s):\nBUS<m>:DPHY:CONFig"}, {"Level"=3, "Class Only"=FALSE, "Identifier"="RSSCOPE_ATTR_PROTOCOL_DPHY_DATA_LANES", "Descriptive Name"="Protocol DPHY Data Lanes", "Data Type"=0, "Command"="BUS{SerialBus}:DPHY:DLAN", "Access"=2, "Range Table"="RsScope_rngDPHYDataLanes", "Read Callback"="", "Write Callback"="", "Supported Models"="", "Instrument Options"="K42", "Flags"=0, "Help"="Sets the number of data lanes. You can select up to four lanes.\n\nAvailable Repeated Capabilities:\nSerialBus: SB1, SB2, SB3, SB4\r\n\nRemote-control command(s):\nBUS<m>:DPHY:DLANes"}, {"Level"=3, "Class Only"=FALSE, "Identifier"="RSSCOPE_ATTR_PROTOCOL_DPHY_CP_SOURCE", "Descriptive Name"="Protocol DPHY CP Source", "Data Type"=0, "Command"="BUS{SerialBus}:DPHY:CP:SOUR", "Access"=2, "Range Table"="rsscope_rngWaveformParameter", "Read Callback"="", "Write Callback"="", "Supported Models"="", "Instrument Options"="K42", "Flags"=0, "Help"="Sets the source of the clock lane.\n\nAvailable Repeated Capabilities:\nSerialBus: SB1, SB2, SB3, SB4\r\n\nRemote-control command(s):\nBUS<m>:DPHY:CP:SOURce"}, {"Level"=3, "Class Only"=FALSE, "Identifier"="RSSCOPE_ATTR_PROTOCOL_DPHY_DN_ZERO_SOURCE", "Descriptive Name"="Protocol DPHY DN Zero Source", "Data Type"=0, "Command"="BUS{SerialBus}:DPHY:DNZ:SOUR", "Access"=2, "Range Table"="rsscope_rngWaveformParameter", "Read Callback"="", "Write Callback"="", "Supported Models"="", "Instrument Options"="K42", "Flags"=0, "Help"="Selects the source of the low power data lanes.\n\nAvailable Repeated Capabilities:\nSerialBus: SB1, SB2, SB3, SB4\r\n\nRemote-control command(s):\nBUS<m>:DPHY:DNZero:SOURce"}, {"Level"=3, "Class Only"=FALSE, "Identifier"="RSSCOPE_ATTR_PROTOCOL_DPHY_DP_ZERO_SOURCE", "Descriptive Name"="Protocol DPHY DP Zero Source", "Data Type"=0, "Command"="BUS{SerialBus}:DPHY:DPZ:SOUR", "Access"=2, "Range Table"="rsscope_rngWaveformParameter", "Read Callback"="", "Write Callback"="", "Supported Models"="", "Instrument Options"="K42", "Flags"=0, "Help"="Selects the source of the low power data lanes.\nThe DP0 lane has to be present all the time, hence Source DP0 > None is not allowed.\n\nAvailable Repeated Capabilities:\nSerialBus: SB1, SB2, SB3, SB4\r\n\nRemote-control command(s):\nBUS<m>:DPHY:DPZero:SOURce"}, {"Level"=3, "Class Only"=FALSE, "Identifier"="RSSCOPE_ATTR_PROTOCOL_DPHY_DP_ONE_SOURCE", "Descriptive Name"="Protocol DPHY DP One Source", "Data Type"=0, "Command"="BUS{SerialBus}:DPHY:DPON:SOUR", "Access"=2, "Range Table"="rsscope_rngWaveformParameter", "Read Callback"="", "Write Callback"="", "Supported Models"="", "Instrument Options"="K42", "Flags"=0, "Help"="Selects the source of the high speed data lane.\n\nAvailable Repeated Capabilities:\nSerialBus: SB1, SB2, SB3, SB4\r\n\nRemote-control command(s):\nBUS<m>:DPHY:DPONe:SOURce"}, {"Level"=3, "Class Only"=FALSE, "Identifier"="RSSCOPE_ATTR_PROTOCOL_DPHY_DP_TWO_SOURCE", "Descriptive Name"="Protocol DPHY DP Two Source", 
